vi "extended result codes.vi"(8 "error in (no error)":errorcluster, 10 "onoff":i32, 11 "para0":dbl) -> (0 "error out":errorcluster, 2 "function return":i32, 3 "para0 out":dbl)   [LabVIEW 2020, in "sqlite3.lvlib"]
uses:
  sqlite3.lvlib
  errstr.vi
  bin/sqlite3_64.dll
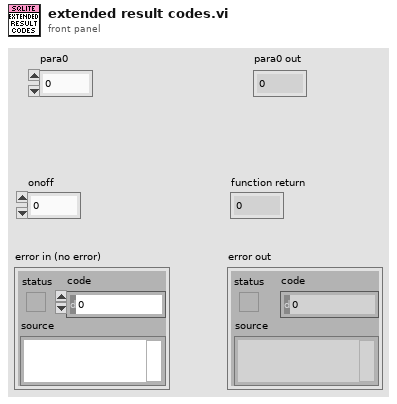
[diagram p1: front panel]
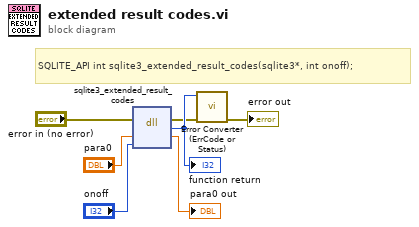
[diagram p0: block diagram]
diagram:
  # "SQLITE_API int sqlite3_extended_result_codes(sqlite3*, int onoff);"
  n1 = dll-call lib="D:/Project/Labview-Projects/database-configuration/externals/sqlite3/Source/bin/sqlite3_*.*" fn="sqlite3_extended_result_codes"(error in="error in (no error)", "para0"="para0", "onoff"="onoff") -> (error out=w2:errorcluster, w7:i32, "para0"=→"para0 out":dbl)  [unwired: 3 in, 1 out]
  "function return" <- w7
  n2 = call "Error Converter (ErrCode or Status).vi"("error in (no error)"=w2, "error code"=w7) -> ("error out"=→"error out":errorcluster)  [unwired: 9 in]
